vi "PathPlanner_Ctrl_LTVUnicyclePack.vi"(4 "Rotation Tolerance DEG":dbl=0.0872665, 6 "Y Tolerance M":dbl=0.0762, 8 "X Tolerance M":dbl=0.0762, 9 "Max Speed M/S":dbl=4.0, 10 "Track Width Meters":dbl=1.0, 11 "LTV_Unicycle_Ctrl_Model":T1={"Max linear ctrl effort M/S"=1.0, "Max angular ctrl effort Rad/S"=2.0, "Max Heading Meas Tol Rad"=0.2, "Max X Pos Meas Tol M"=0.0625, "Max Y Pos Meas Tol M"=0.125, "Max Linear Vel M/S"=9.0} {"Max Linear Vel M/S" format="%#_13g"; "Max Y Pos Meas Tol M" format="%#_13g"; "Max X Pos Meas Tol M" format="%#_13g"; "Max Heading Meas Tol Rad" format="%#_13g"; "Max angular ctrl effort Rad/S" format="%#_13g"; "Max linear ctrl effort M/S" format="%#_13g"}) -> (3 "PathPlanner_Ctrl_LTVUnicycleConfig":T2={"Max Wheel Speed M/S"=0.0, "Track Width M"=0.0, "LTV_Unicycle_Ctrl_Model"={"Max linear ctrl effort M/S"=0.0, "Max angular ctrl effort Rad/S"=0.0, "Max Heading Meas Tol Rad"=0.0, "Max X Pos Meas Tol M"=9.9e+30, "Max Y Pos Meas Tol M"=-9.9e+30, "Max Linear Vel M/S"=0.0}, "LTV_Unicycle_Ctrl_Tolerance"={"Max Heading Tolerance Rad"=0.0, "Max X Tolerance M"=0.0, "Max Y Tolerance M"=9.9e+30}} {"LTV_Unicycle_Ctrl_Tolerance"."Max Y Tolerance M" format="%#_13g"; "LTV_Unicycle_Ctrl_Tolerance"."Max X Tolerance M" format="%#_13g"; "LTV_Unicycle_Ctrl_Tolerance"."Max Heading Tolerance Rad" format="%#_13g"; "LTV_Unicycle_Ctrl_Model"."Max Linear Vel M/S" format="%#_13g"; "LTV_Unicycle_Ctrl_Model"."Max Y Pos Meas Tol M" format="%#_13g"; "LTV_Unicycle_Ctrl_Model"."Max X Pos Meas Tol M" format="%#_13g"; "LTV_Unicycle_Ctrl_Model"."Max Heading Meas Tol Rad" format="%#_13g"; "LTV_Unicycle_Ctrl_Model"."Max angular ctrl effort Rad/S" format="%#_13g"; "LTV_Unicycle_Ctrl_Model"."Max linear ctrl effort M/S" format="%#_13g"})   [LabVIEW 2019, in "PathPlanner24.lvlib"]
doc: "Pack controller tuning configuration for Differential Drive LTV Unicycle Controller.\n\nInputs:\n - LTV_Unicycle_Ctrl_Model - cluster - The modeling paraameters for the LTV drive controller. These are static. They should not be changed after the first call to this function.\n - Track With - double - Track width (Meters)\n - Max Wheel Speed M/.S - double - Maximum wheel speed (M/S)\n - X Tolerance -- X tolerance for calculating At Reference (Meters) (Optional. Default: 0.0762 )\n - Y Tolerance -- Y tolerance for calculating At Reference (Meters) (Optional. Default: 0.0762 )\n - Rotation Tolerance -- Rotation tolerance for calculating At Reference (Degrees) (Optional. Default: 0.0)873)\n\nOutputs:\n -- PathPlannerLTVUnicycleCtrlConfig -- cluster - packed controller configuration."
uses:
  PathPlanner24.lvlib
  TypeDef/PathPlannerCtrlLTVUnicycleConfig.ctl
  <vilib>/Rock Robotics/WPI/ThirdParty/JAS_Junk/TrajLib/TypeDef/LTV_UNICYCLE_CONTROLLER_MODEL_PARAMS.CTL
  <vilib>/Rock Robotics/WPI/ThirdParty/JAS_Junk/TrajLib/TypeDef/LTV_UNICYCLE_CONTROLLER_TOLERANCE.CTL
  <vilib>/Rock Robotics/WPI/ThirdParty/JAS_Junk/TrajLib/Trajectory_Library.lvlib
panel:
  # "3 inches"
  # "5 deg"
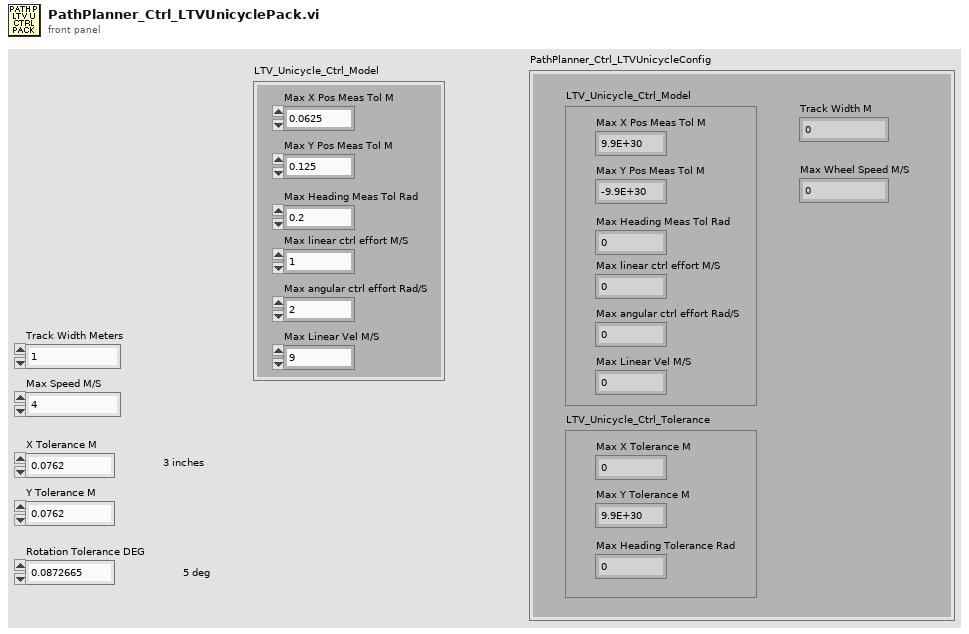
[diagram p1: front panel]
types:
  T1 = typedef "Trajectory_Library.lvlib/LTV_UNICYCLE_CONTROLLER_MODEL_PARAMS.CTL" = cluster{"Max linear ctrl effort M/S":dbl, "Max angular ctrl effort Rad/S":dbl, "Max Heading Meas Tol Rad":dbl, "Max X Pos Meas Tol M":dbl, "Max Y Pos Meas Tol M":dbl, "Max Linear Vel M/S":dbl}
  T2 = typedef "PathPlanner24.lvlib/PathPlannerCtrlLTVUnicycleConfig.ctl" = cluster{"Max Wheel Speed M/S":dbl, "Track Width M":dbl, "LTV_Unicycle_Ctrl_Model":T1, "LTV_Unicycle_Ctrl_Tolerance":T3}
  T3 = typedef "Trajectory_Library.lvlib/LTV_UNICYCLE_CONTROLLER_TOLERANCE.CTL" = cluster{"Max Heading Tolerance Rad":dbl, "Max X Tolerance M":dbl, "Max Y Tolerance M":dbl}
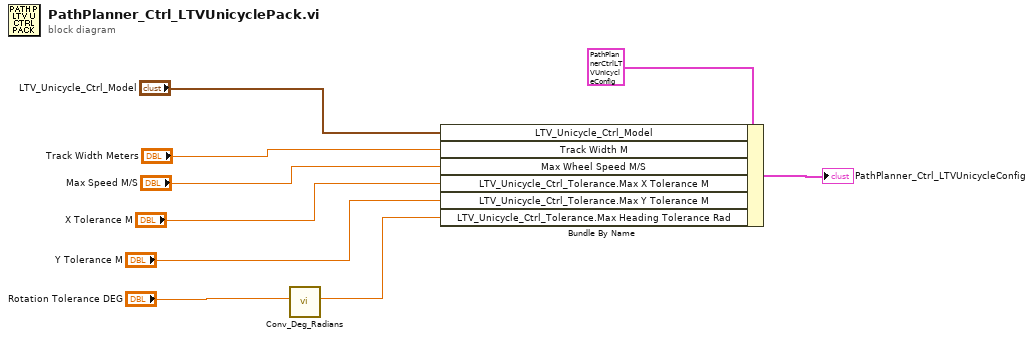
[diagram p0: block diagram]
diagram:
  n1 = call <vilib>:"Conv_Deg_Radians.vi"("Degress"="Rotation Tolerance DEG") -> ("Radians"=w1:dbl)  [unwired: 10 in]
  n2 = Bundle By Name(cluster=T2 {"Max Wheel Speed M/S"=0.0, "Track Width M"=0.0, "LTV_Unicycle_Ctrl_Model"={"Max linear ctrl effort M/S"=1.0, "Max angular ctrl effort Rad/S"=2.0, "Max Heading Meas Tol Rad"=0.2, "Max X Pos Meas Tol M"=0.0625, "Max Y Pos Meas Tol M"=0.125, "Max Linear Vel M/S"=9.0}, "LTV_Unicycle_Ctrl_Tolerance"={"Max Heading Tolerance Rad"=1.0, "Max X Tolerance M"=2.0, "Max Y Tolerance M"=0.2}} ("PathPlanner_Ctrl_LTVUnicycle_Config"), "LTV_Unicycle_Ctrl_Model"="LTV_Unicycle_Ctrl_Model", "Track Width M"="Track Width Meters", "Max Wheel Speed M/S"="Max Speed M/S", "LTV_Unicycle_Ctrl_Tolerance.Max X Tolerance M"="X Tolerance M", "LTV_Unicycle_Ctrl_Tolerance.Max Y Tolerance M"="Y Tolerance M", "LTV_Unicycle_Ctrl_Tolerance.Max Heading Tolerance Rad"=w1) -> (→"PathPlanner_Ctrl_LTVUnicycleConfig":T2)
